vi "prep8742 (SubVI).vi"(7 "error in (no error)":errorcluster, 9 "DeviceKey Out in":string, 10 ".NET Refnum in":refnum<k24>) -> (0 "error out":errorcluster, 1 "DeviceKey Out out":string, 2 "Device Address Out":i32, 3 ".NET Refnum out":refnum<k24>)   [LabVIEW 2019]
uses:
  C:/Users/jyxks/OneDrive/Documents/Program Files/New Focus/New Focus Picomotor Application/Samples/LabVIEW/Model 8742/LabVIEW 2009/CmdLib.dll
  Program Files/New Focus/New Focus Picomotor Application/Samples/LabVIEW/Model 8742/LabVIEW 2009/CmdLib.dll
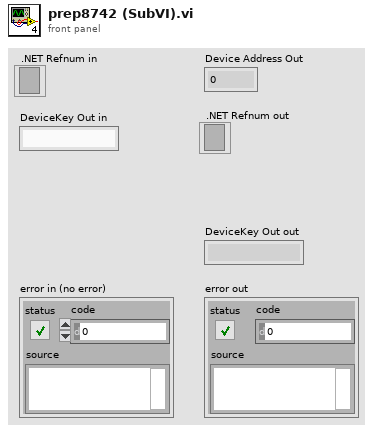
[diagram p1: front panel]
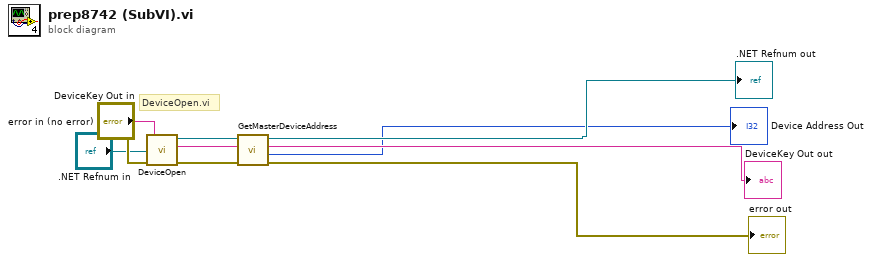
[diagram p0: block diagram]
diagram:
  # "DeviceOpen.vi"
  n1 = call "DeviceOpen.vi"("error in (no error)"="error in (no error)", "DeviceKey In"="DeviceKey Out in", "CmdLib In"=".NET Refnum in") -> ("error out"=w10:errorcluster, "DeviceKey Out"=w9:string, "CmdLib Out"=w8:refnum<k24>)  [unwired: 2 in]
  n2 = call "GetMasterDeviceAddress.vi"("error in (no error)"=w10, "DeviceKey In"=w9, "CmdLib In"=w8) -> ("error out"=→"error out":errorcluster, "Device Address"=→"Device Address Out":i32, "DeviceKey Out"=→"DeviceKey Out out":string, "CmdLib Out"=→".NET Refnum out":refnum<k24>)  [unwired: 1 in]
